vi "assembleProjections.vi"(6 "calc ff/fb":bool, 7 "tracking":bool, 8 "error in (no error)":errorcluster, 10 "Queues":T5) -> (0 "error out":errorcluster, 2 "sample volume to assemble":T1, 5 "status":T4)   [LabVIEW 2010]
uses:
  internal_queues.ctl
  line_info.ctl
  volume_with_lines.ctl
  volume_info.ctl
  kalman_result_scaled.ctl
  projection buffers.ctl
  location3D.ctl
  spot location.ctl
  addLineToProjections.vi
  get write location projection.vi
  sum line into array.vi
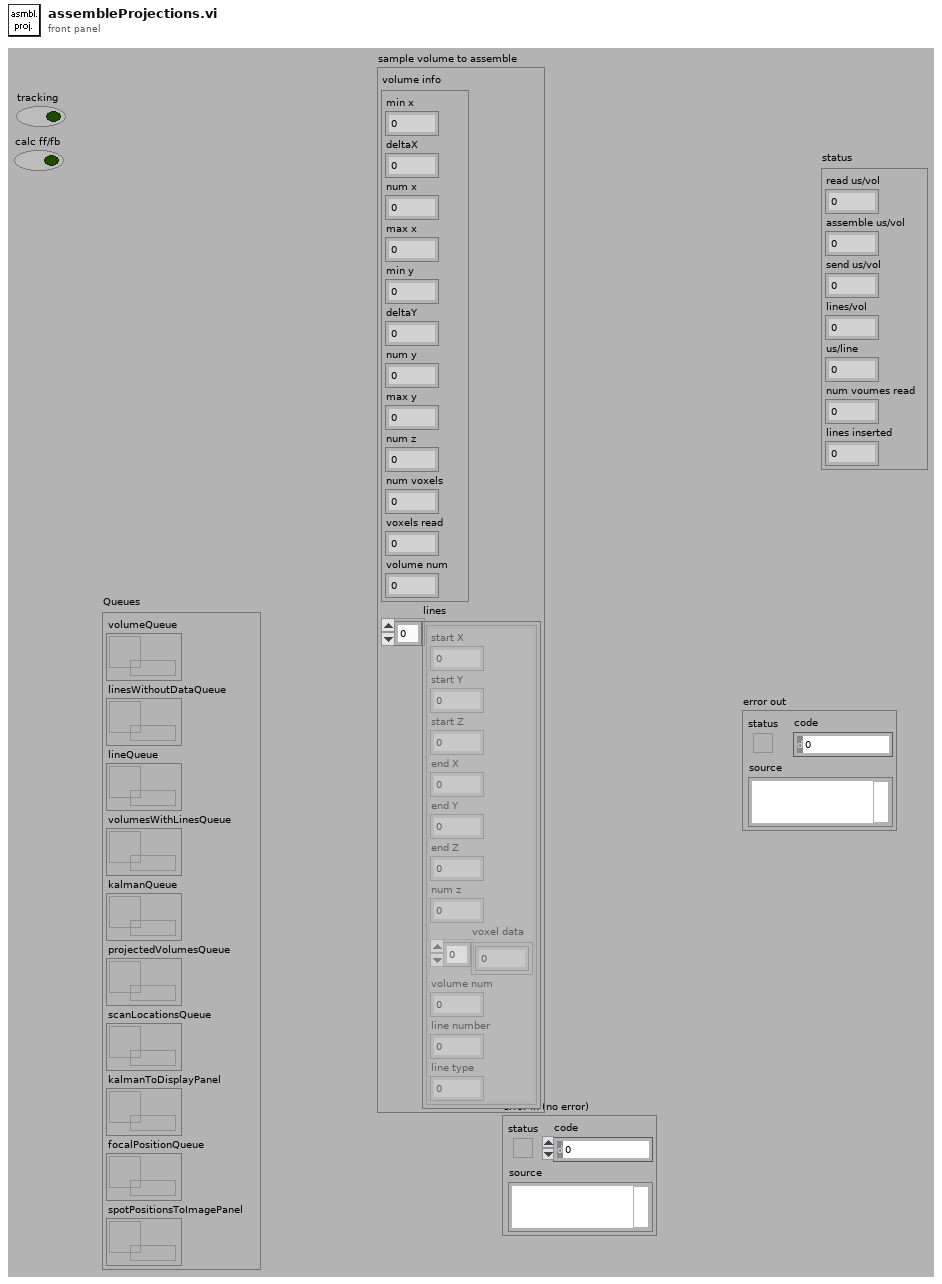
[diagram p1: front panel]
types:
  T1 = typedef "volume_with_lines.ctl" = cluster{"volume info":T2, "lines":T3[]}
  T2 = typedef "volume_info.ctl" = cluster{"min x":i16, "deltaX":dbl, "num x":u32, "max x":i16, "min y":i16, "deltaY":dbl, "num y":u32, "max y":i16, "num z":u32, "num voxels":u32, "voxels read":u32, "volume num":u32}
  T3 = typedef "line_info.ctl" = cluster{"start X":i16, "start Y":i16, "start Z":i16, "end X":i16, "end Y":i16, "end Z":i16, "num z":u8, "voxel data":u32[], "volume num":u32, "line number":u16, "line type":u16}
  T4 = cluster{"read us/vol":dbl, "assemble us/vol":dbl, "send us/vol":dbl, "lines/vol":dbl, "us/line":dbl, "num voumes read":u32, "lines inserted":i32}
  T5 = typedef "internal_queues.ctl" = cluster{"volumeQueue":refnum<queue>, "linesWithoutDataQueue":refnum<queue>, "lineQueue":refnum<queue>, "volumesWithLinesQueue":refnum<queue>, "kalmanQueue":refnum<queue>, "projectedVolumesQueue":refnum<queue>, "scanLocationsQueue":refnum<queue>, "kalmanToDisplayPanel":refnum<queue>, "focalPositionQueue":refnum<queue>, "spotPositionsToImagePanel":refnum<queue>}
  T6 = typedef "projection buffers.ctl" = cluster{"xy buffer":u32[], "zx buffer":u32[], "zy buffer":u32[], "zx buffer fb only":u32[], "zy buffer fb only":u32[]}
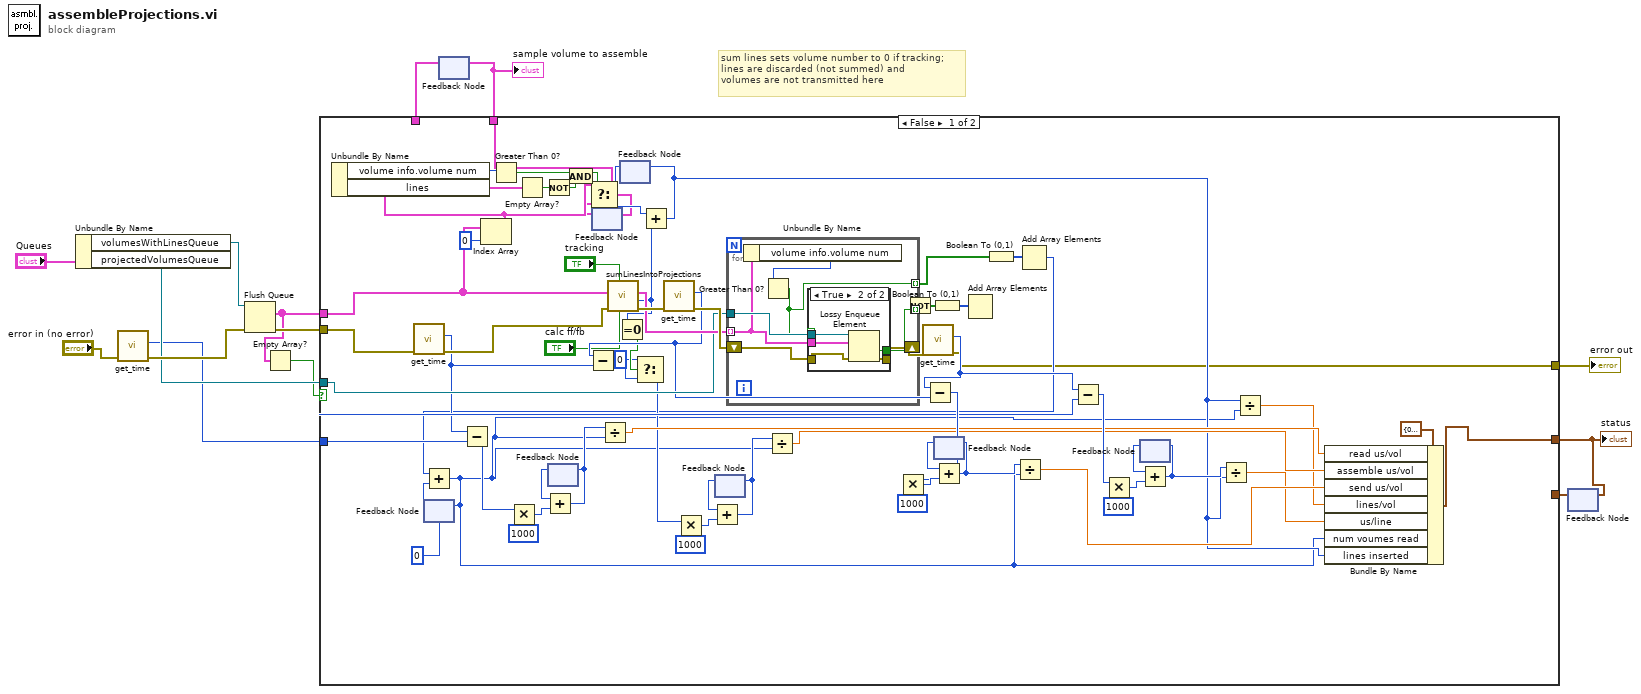
[diagram p0: block diagram]
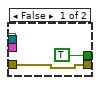
[diagram p2: hidden frame]
diagram:
  # "sum lines sets volume number to 0 if tracking;\nlines are discarded (not summed) and\nvolumes are not transmitted here"
  n1 = Unbundle By Name("Queues") -> ("volumesWithLinesQueue"=w14:refnum<queue>, "projectedVolumesQueue"=w11:refnum<queue>)
  n2 = call "get_time.vi"("error in (no error)"="error in (no error)") -> ("error out"=w12:errorcluster, "millisecond timer value"=w10:u32)  [unwired: 9 in]
  n3 = Flush Queue(queue=w14, error in (no error)=w12) -> (remaining elements=w7:T1[], error out=w9:errorcluster)  [unwired: 1 out]
  n4 = Empty Array?(array=w7) -> (empty?=w6:bool)
  n5 = feedback #1() -> (w1:T1)  [unwired: 1 in]
  n6 = feedback #2() -> (w4:T4)  [unwired: 1 in]
  n7 = case shown="False" w6 {
    tunnel: w11 -> [w74 _]
    tunnel: w10 -> [w54 _]
    tunnel: w9 -> [w48 w97]
    tunnel: w7 -> [w25 _]
    tunnel: [w34 w98] -> w5
    tunnel: w4 -> [_ w98]
    tunnel: [w30 w97] -> w3
    tunnel: [w19 w96] -> w2
    tunnel: w1 -> [_ w96]
    frame False {
      n8 = call "get_time.vi"("error in (no error)"=w48) -> ("error out"=w47:errorcluster, "millisecond timer value"=w42:u32)  [unwired: 9 in]
      n9 = feedback #3(0) -> (w69:i32)
      n10 = Subtract(x=w42, y=w54) -> (x-y=w67:u32)
      n11 = Index Array(array=w25, index=0) -> (element=w21:T1)
      n12 = Unbundle By Name(w21) -> ("volume info.volume num"=w23:u32, "lines"=w18:T3[])
      n13 = Greater Than 0?(x=w23) -> (x > 0?=w22:bool)
      n14 = Multiply(x=w67, y=u32 1000 ("x")) -> (x*y=w80:u32)
      n15 = Empty Array?(array=w18) -> (empty?=w17:bool)
      n16 = Not(x=w17) -> (.not. x?=w15:bool)
      n17 = feedback #4() -> (w79:u32)  [unwired: 1 in]
      n18 = Add(x=w79, y=w80) -> (x+y=w78:u32)
      n19 = feedback-in #4(w78) -> ()
      n20 = And(x=w22, y=w15) -> (x .and. y?=w16:bool)
      n21 = feedback #5() -> (w20:T1)  [unwired: 1 in]
      n22 = Select(t=w21, s=w16, f=w20) -> (s? t:f=w19:T1)
      n23 = feedback-in #5(w19) -> ()
      n24 = call "sumLinesIntoProjections.vi"("calc ff/fb"="calc ff/fb", "tracking"="tracking", "error in (no error)"=w47, "volumes to assemble"=w25) -> ("error out"=w77:errorcluster, "lines inserted"=w39:i32, "volumes to send"=w75:cluster{"volume info":T2, "buffers":T6}[])  [unwired: 5 in]
      n25 = Equal To 0?(x=w39) -> (x = 0?=w38:bool)
      n26 = feedback #6() -> (w46:i32)  [unwired: 1 in]
      n27 = Add(x=w46, y=w39) -> (x+y=w33:i32)
      n28 = feedback-in #6(w33) -> ()
      n29 = call "get_time.vi"("error in (no error)"=w77) -> ("error out"=w76:errorcluster, "millisecond timer value"=w57:u32)  [unwired: 9 in]
      n30 = Subtract(x=w57, y=w42) -> (x-y=w63:u32)
      n31 = Select(t=u32 0, s=w38, f=w63) -> (s? t:f=w40:u32)
      n32 = Multiply(x=w40, y=u32 1000 ("x")) -> (x*y=w65:u32)
      n33 = feedback #7() -> (w64:u32)  [unwired: 1 in]
      n34 = Add(x=w64, y=w65) -> (x+y=w62:u32)
      n35 = feedback-in #7(w62) -> ()
      n36 = for {
        tunnel: w75 -> [w84] mode=indexing
        tunnel: w74 -> [w88]
        shift-right: [w87] -> w70
        shift-left: w76 -> [w85]
        tunnel: [w86] -> w73 mode=indexing
        tunnel: [w82] -> w29 mode=indexing
        n37 = Unbundle By Name(w84) -> ("volume info.volume num"=w83:u32)
        n38 = Greater Than 0?(x=w83) -> (x > 0?=w82:bool)
        n39 = case shown="True" w82 {
          tunnel: w88 -> [_ w95]
          tunnel: [w89 w94] -> w87
          tunnel: [TRUE ("overflow?") w93] -> w86
          tunnel: w85 -> [w89 w92]
          tunnel: w84 -> [_ w91]
          frame False {
          }
          frame True {
            n40 = Lossy Enqueue Element(queue=w95, element=w91, error in (no error)=w92) -> (overflow?=w93:bool, error out=w94:errorcluster)  [unwired: 2 out]
          }
        }
      }
      n41 = Not(x=w73) -> (.not. x?=w72:bool[])
      n42 = call "get_time.vi"("error in (no error)"=w70) -> ("error out"=w30:errorcluster, "millisecond timer value"=w55:u32)  [unwired: 9 in]
      n43 = Subtract(x=w55, y=w57) -> (x-y=w56:u32)
      n44 = Multiply(x=w56, y=u32 1000 ("x")) -> (x*y=w61:u32)
      n45 = Boolean To (0,1)(Boolean=w72) -> (0, 1=w71:i16[])
      n46 = feedback #8() -> (w60:u32)  [unwired: 1 in]
      n47 = Add(x=w60, y=w61) -> (x+y=w58:u32)
      n48 = feedback-in #8(w58) -> ()
      n49 = Add Array Elements(numeric array=w71) -> ()  [unwired: 1 out]
      n50 = Boolean To (0,1)(Boolean=w29) -> (0, 1=w44:i16[])
      n51 = Add Array Elements(numeric array=w44) -> (sum=w32:i16)
      n52 = Add(x=w32, y=w69) -> (x+y=w28:i32)
      n53 = feedback-in #3(w28) -> ()
      n54 = Divide(x=w78, y=w28) -> (x/y=w43:dbl)
      n55 = Divide(x=w62, y=w28) -> (x/y=w41:dbl)
      n56 = Divide(x=w58, y=w28) -> (x/y=w36:dbl)
      n57 = Subtract(x=w55, y=w54) -> (x-y=w49:u32)
      n58 = Multiply(x=w49, y=u32 1000 ("x")) -> (x*y=w53:u32)
      n59 = feedback #9() -> (w52:u32)  [unwired: 1 in]
      n60 = Add(x=w52, y=w53) -> (x+y=w50:u32)
      n61 = feedback-in #9(w50) -> ()
      n62 = Divide(x=w50, y=w33) -> (x/y=w35:dbl)
      n63 = Divide(x=w33, y=w28) -> (x/y=w31:dbl)
      n64 = Bundle By Name(cluster=T4 {"read us/vol"=0.0, "assemble us/vol"=0.0, "send us/vol"=0.0, "lines/vol"=0.0, "us/line"=0.0, "num voumes read"=0, "lines inserted"=0} ("status"), "read us/vol"=w43, "assemble us/vol"=w41, "send us/vol"=w36, "lines/vol"=w31, "us/line"=w35, "num voumes read"=w28, "lines inserted"=w33) -> (w34:T4)
    }
    frame True {
    }
  }
  "status" <- w5
  "error out" <- w3
  "sample volume to assemble" <- w2
  n65 = feedback-in #1(w2) -> ()
  n66 = feedback-in #2(w5) -> ()
